vi "Process Insert Assert.vi"(6 "Wire UID":i32, 7 "Assert Add Configuration":T1, 8 "error in (no error)":errorcluster, 9 "appended path":path, 10 "Wire ref in":refnum<vi>, 11 "Caller VI Reference":refnum<vi>) -> (0 "error out":errorcluster)   [LabVIEW 2018]
doc: "Queued state machine to allow an assert to be added into the calling vi correctly based on the configuration set. This requires operations to execute in different orders"
uses:
  Assert Add Configuration.ctl
  Insert Process Data.ctl
  <vilib>/Utility/error.llb/Error Cluster From Error Code.vi
  <vilib>/ErrorRing/Error Ring.xnode
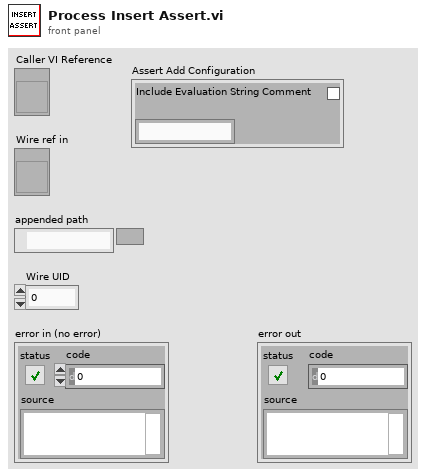
[diagram p1: front panel]
types:
  T1 = typedef "Assert Add Configuration.ctl" = cluster{"Include Evaluation String Comment":bool, "Eval String":string}
  T2 = typedef "Insert Process Data.ctl" = cluster{"Wire Ref":refnum<vi>, "Assert VI Instance Ref":refnum<vi>, "Assert VI Path":path, "Caller VI Ref":refnum<vi>, "Temp VI Path":path}
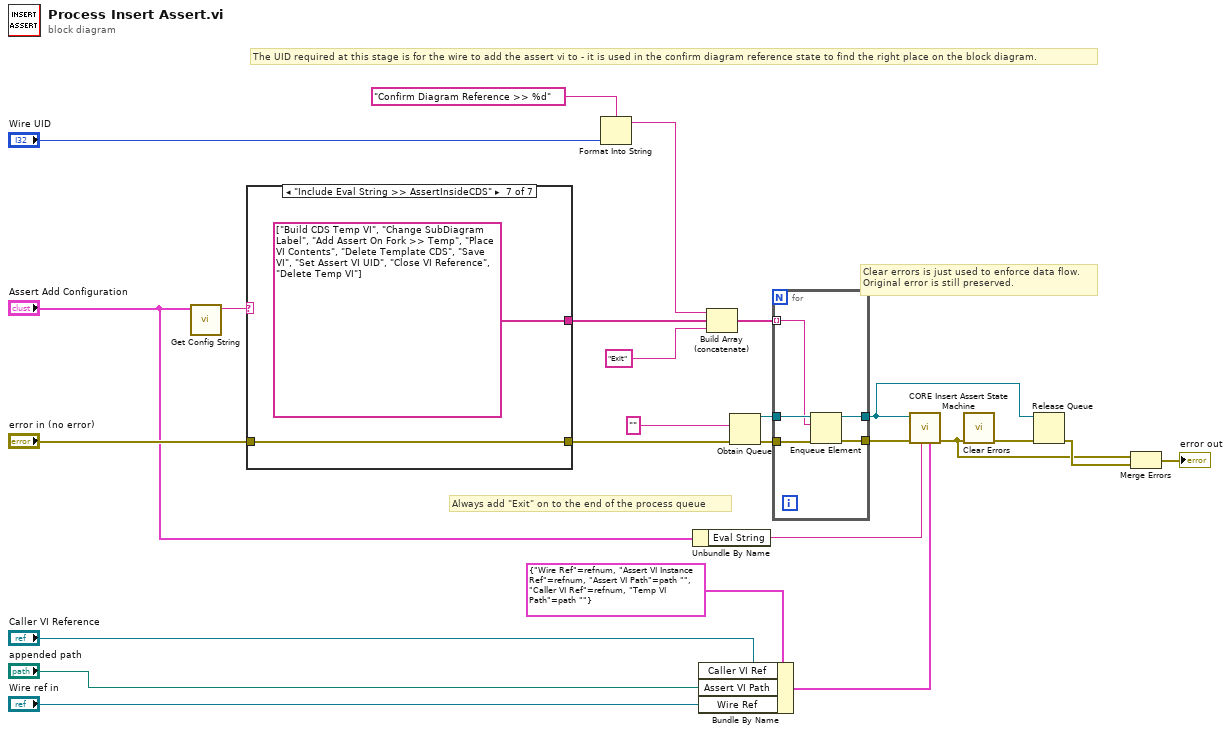
[diagram p0: block diagram]
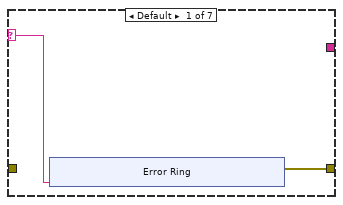
[diagram p2: hidden frame]
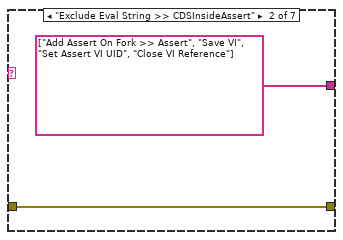
[diagram p3: hidden frame]
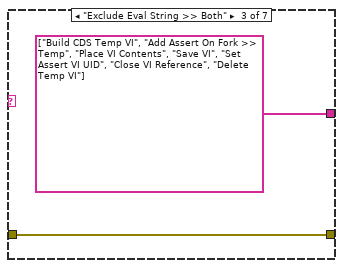
[diagram p4: hidden frame]
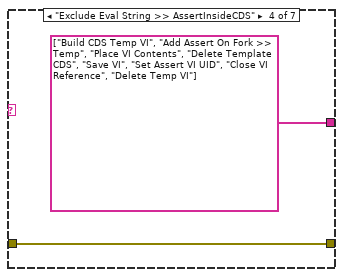
[diagram p5: hidden frame]
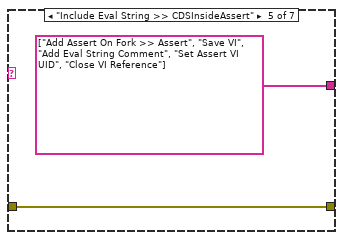
[diagram p6: hidden frame]
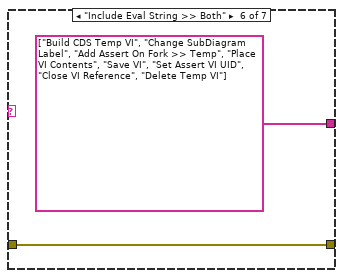
[diagram p7: hidden frame]
diagram:
  # "Clear errors is just used to enforce data flow.\nOriginal error is still preserved."
  # "The UID required at this stage is for the wire to add the assert vi to - it is used in the confirm diagram reference state to find the right place on the block diagram."
  # "Always add \"Exit\" on to the end of the process queue"
  n1 = call "Get Config String.vi"("Assert Add Configuration"="Assert Add Configuration") -> ("Case"=w15:string)  [unwired: 10 in]
  n2 = case shown="\"Include Eval String >> AssertInsideCDS\"" w15 {
    selector: w15 -> [w27 _ _ _ _ _ _]
    tunnel: [_ string[] ["Add Assert On Fork >> Assert", "Save VI", "Set Assert VI UID", "Close VI Reference"] string[] ["Build CDS Temp VI", "Add Assert On Fork >> Temp", "Place VI Contents", "Save VI", "Set Assert VI UID", "Close VI Reference", "Delete Temp VI"] string[] ["Build CDS Temp VI", "Add Assert On Fork >> Temp", "Place VI Contents", "Delete Template CDS", "Save VI", "Set Assert VI UID", "Close VI Reference", "Delete Temp VI"] string[] ["Add Assert On Fork >> Assert", "Save VI", "Add Eval String Comment", "Set Assert VI UID", "Close VI Reference"] string[] ["Build CDS Temp VI", "Change SubDiagram Label", "Add Assert On Fork >> Temp", "Place VI Contents", "Save VI", "Set Assert VI UID", "Close VI Reference", "Delete Temp VI"] string[] ["Build CDS Temp VI", "Change SubDiagram Label", "Add Assert On Fork >> Temp", "Place VI Contents", "Delete Template CDS", "Save VI", "Set Assert VI UID", "Close VI Reference", "Delete Temp VI"]] -> w9
    tunnel: "error in (no error)" -> [_ w35 w37 w39 w41 w43 w45]
    tunnel: [w26 w35 w37 w39 w41 w43 w45] -> w13
    frame Default {
      n3 = xnode "Error Ring"("parameter 0"=w27) -> ("error out"=w26:errorcluster)
    }
    frame "Exclude Eval String >> CDSInsideAssert" {
    }
    frame "Exclude Eval String >> Both" {
    }
    frame "Exclude Eval String >> AssertInsideCDS" {
    }
    frame "Include Eval String >> CDSInsideAssert" {
    }
    frame "Include Eval String >> Both" {
    }
    frame "Include Eval String >> AssertInsideCDS" {
    }
  }
  n4 = Format Into String(format string="Confirm Diagram Reference >> %d" ("String"), "Wire UID") -> (resulting string=w6:string)  [unwired: 2 in, 1 out]
  n5 = Unbundle By Name("Assert Add Configuration") -> ("Eval String"=w2:string)
  n6 = Bundle By Name(cluster=T2 {"Wire Ref"=refnum, "Assert VI Instance Ref"=refnum, "Assert VI Path"=path "", "Caller VI Ref"=refnum, "Temp VI Path"=path ""}, "Caller VI Ref"="Caller VI Reference", "Assert VI Path"="appended path", "Wire Ref"="Wire ref in") -> (w1:T2)
  n7 = Build Array (concatenate)(w6, w9, "Exit" ("String")) -> (w11:string[])
  n8 = Obtain Queue(element data type="", error in (no error)=w13) -> (queue out=w24:refnum<queue>, error out=w23:errorcluster)  [unwired: 3 in, 1 out]
  n9 = for {
    tunnel: w24 -> [w51]
    tunnel: w23 -> [w50]
    tunnel: w11 -> [w49] mode=indexing
    tunnel: [w48] -> w5
    tunnel: [w47] -> w22
    n10 = Enqueue Element(queue=w51, element=w49, error in (no error)=w50) -> (queue out=w48:refnum<queue>, error out=w47:errorcluster)  [unwired: 1 in, 1 out]
  }
  n11 = call "CORE Insert Assert State Machine.vi"("Cluster"=w1, "Eval String"=w2, "error in (no error)"=w22, "Queue in"=w5) -> ("error out"=w4:errorcluster)  [unwired: 7 in]
  n12 = call <vilib>:"Clear Errors.vi"("error in (no error)"=w4) -> ("error out"=w3:errorcluster)  [unwired: 5 in, 1 out]
  n13 = Release Queue(queue=w5, error in (no error)=w3) -> (error out=w21:errorcluster)  [unwired: 1 in, 2 out]
  n14 = Merge Errors(w4, w21) -> (→"error out":errorcluster)
